vi "FMDLWriteHeaderLineToMeasurementFile.vi"(0 "Refnum in":refnum<file>, 1 "Spacer Line?":bool, 2 "Header Key String":string, 3 "Header Value Number":dbl, 4 "Header Value String":string, 5 "error in (no error)":errorcluster) -> (6 "refnum out":refnum<file>, 7 "Comment character":string="%", 8 "error out":errorcluster)   [LabVIEW 2018]
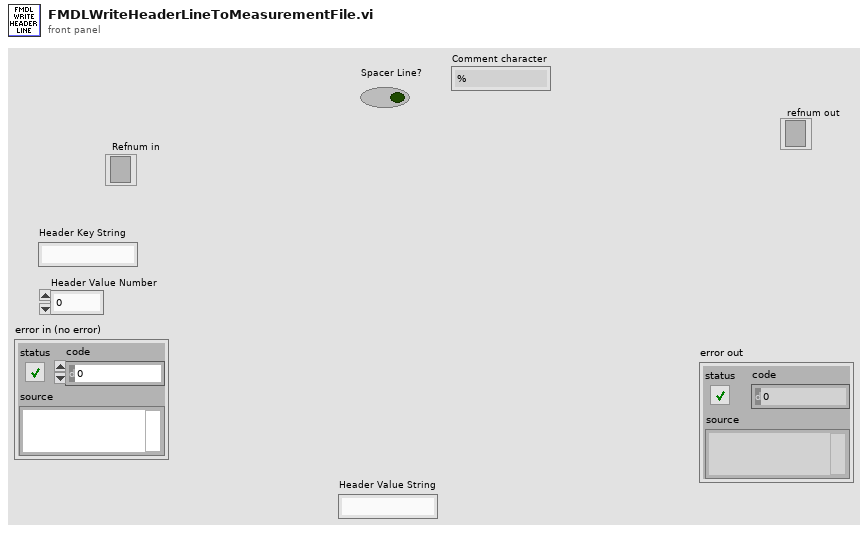
[diagram p1: front panel]
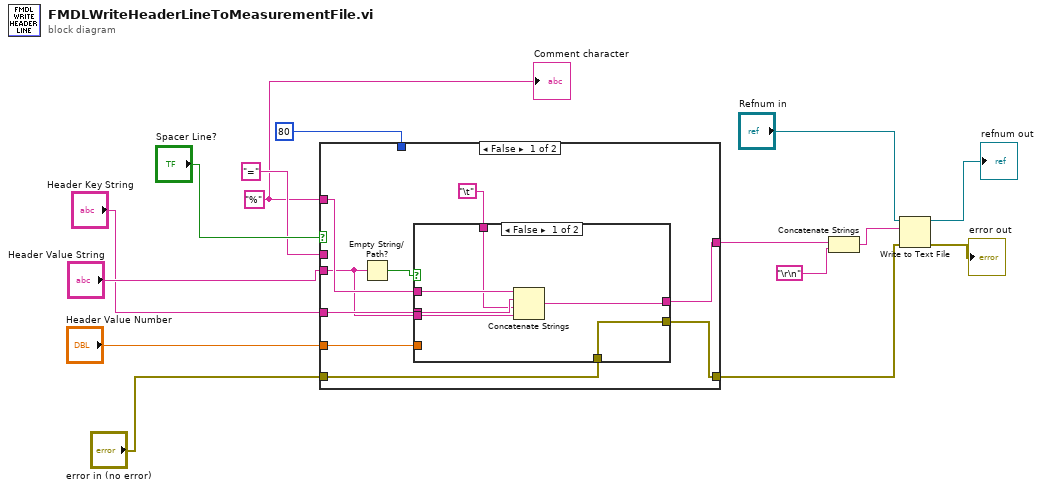
[diagram p0: block diagram]
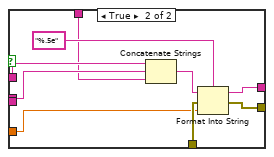
[diagram p2: hidden frame]
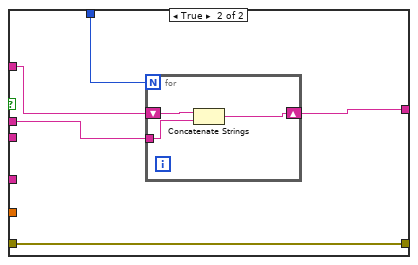
[diagram p3: hidden frame]
diagram:
  w8 = "%"
  n1 = case shown="False" "Spacer Line?" {
    tunnel: 80 -> [_ w44]
    tunnel: "=" -> [_ w40]
    tunnel: [w18 w43] -> w4
    tunnel: "error in (no error)" -> [w21 w42]
    tunnel: [w20 w42] -> w11
    tunnel: w8 -> [w23 w41]
    tunnel: "Header Value String" -> [w16 _]
    tunnel: "Header Key String" -> [w22 _]
    tunnel: "Header Value Number" -> [w19 _]
    frame False {
      n2 = Empty String/Path?(string/path=w16) -> (empty?=w24:bool)
      n3 = case shown="False" w24 {
        tunnel: w23 -> [w30 w39]
        tunnel: w22 -> [w29 w38]
        tunnel: w21 -> [w25 w35]
        tunnel: [w25 w34] -> w20
        tunnel: w19 -> [_ w33]
        tunnel: [w26 w32] -> w18
        tunnel: "\t" -> [w28 w31]
        tunnel: w16 -> [w27 _]
        frame False {
          n4 = Concatenate Strings(w30, w29, w28, w27) -> (w26:string)
        }
        frame True {
          n5 = Concatenate Strings(w39, w38, w31) -> (w36:string)
          n6 = Format Into String(format string="%.5e", initial string=w36, error in=w35, w33) -> (resulting string=w32:string, error out=w34:errorcluster)
        }
      }
    }
    frame True {
      n7 = for {
        N: w44 -> [_]
        shift-right: [w45] -> w43
        shift-left: w41 -> [w47]
        tunnel: w40 -> [w46]
        n8 = Concatenate Strings(w47, w46) -> (w45:string)
      }
    }
  }
  n9 = Concatenate Strings(w4, "\r\n") -> (w2:string)
  n10 = Write to Text File(file (use dialog)="Refnum in", text=w2, error in=w11) -> (refnum out=→"refnum out":refnum<file>, error out=→"error out":errorcluster)  [unwired: 1 in, 1 out]
  "Comment character" <- w8
